vi "Write System State.vi"(8 "error in (no error)":errorcluster, 10 "System State":T1, 11 "DROPBEAR_Model_Updating in":refnum<class "DROPBEAR_Model_Updating.lvclass">) -> (0 "error out":errorcluster, 3 "DROPBEAR_Model_Updating out":refnum<class "DROPBEAR_Model_Updating.lvclass">)   [LabVIEW 2021, in "DROPBEAR_Model_Updating.lvclass"]
uses:
  DROPBEAR_Model_Updating.lvclass
  DROPBEAR_Model_Updating.lvclass/DROPBEAR_Model_Updating.ctl
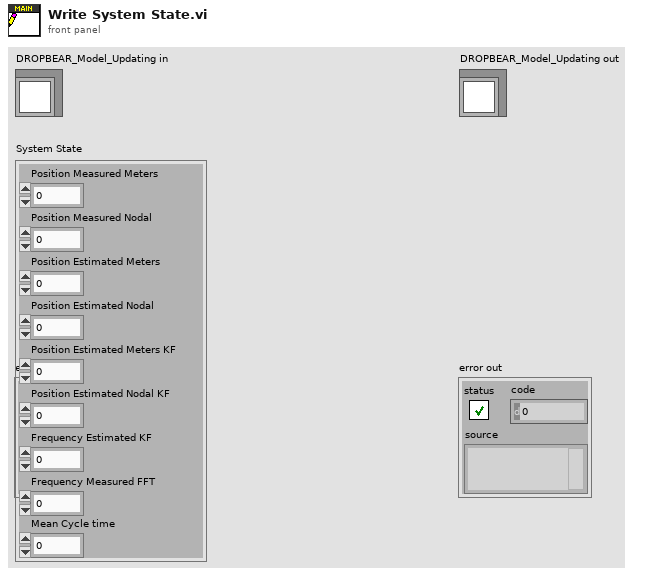
[diagram p1: front panel]
types:
  T1 = cluster{"Position Measured Meters":dbl, "Position Measured Nodal":i32, "Position Estimated Meters":dbl, "Position Estimated Nodal":i32, "Frequency Estimated KF":dbl, "Frequency Measured FFT":dbl, "Position Estimated Meters KF":dbl, "Position Estimated Nodal KF":i32, "Mean Cycle time":dbl}
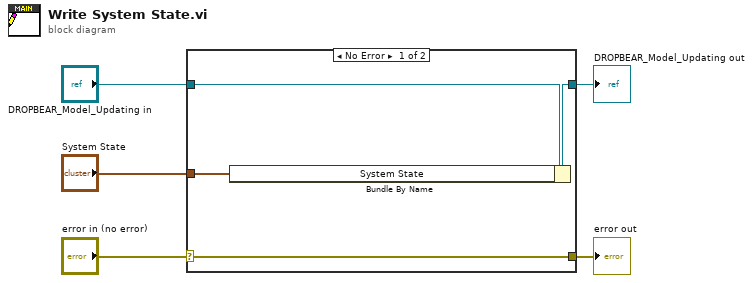
[diagram p0: block diagram]
diagram:
  n1 = case shown="No Error" "error in (no error)" {
    selector: "error in (no error)" -> [w9 w10]
    tunnel: [w9 w10] -> w4
    tunnel: [w7 w11] -> w2
    tunnel: "DROPBEAR_Model_Updating in" -> [w8 w11]
    tunnel: "System State" -> [w6 _]
    frame No Error {
      n2 = Bundle By Name(cluster=w8, "System State"=w6) -> (w7:refnum<class "DROPBEAR_Model_Updating.lvclass">)
    }
    frame Error {
    }
  }
  "error out" <- w4
  "DROPBEAR_Model_Updating out" <- w2
